vi "UTIL Temp Control.vi"(3 "Evaluate":bool, 4 "Parameters In":dbl[](array[numeric]), 5 "Class":i32) -> (1 "Parameters Out":dbl[](array[numeric]))   [LabVIEW 2010]
doc: "This VI keeps track of the number of Sleep and Wake classifications over a desired interval, and modifies the target ambient temperature based on the sleep-wake ratio. It stores 5 values in a shift register (Parameters In/Out):\n1. Error (Q - Q*)\n2. Target Temperature\n3. Sleep Count\n4. Wake Count\n5. Previous Temperature Change\n\nInputs: \n Class SGL, predicted sleep stage\n Parameters In 1-D Array of Double\n Evaluate Boolean, true at end of time period\nOutputs:\n Parameters Out 1-D Array of DBL"
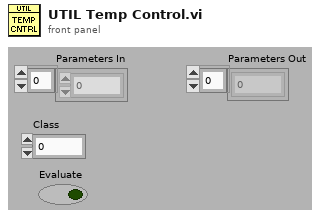
[diagram p1: front panel]
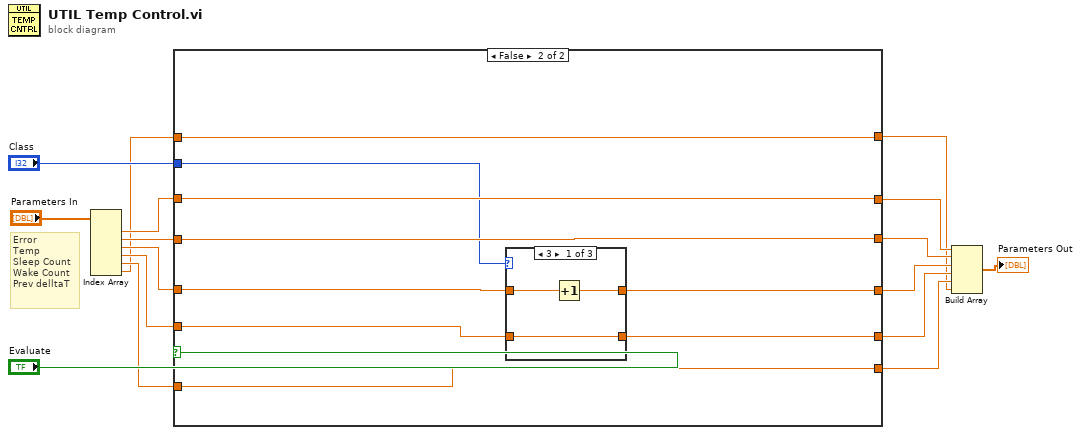
[diagram p0: block diagram]
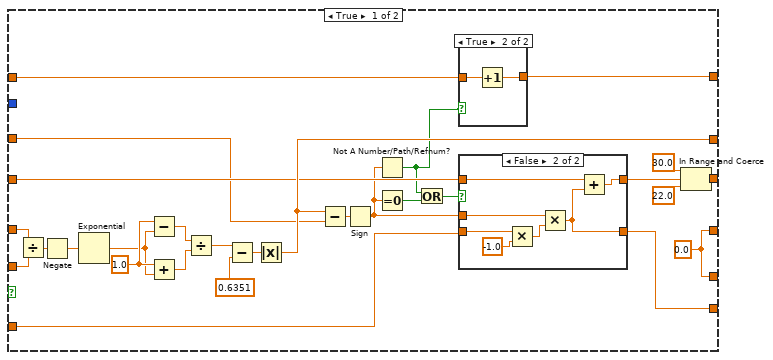
[diagram p2: hidden frame]
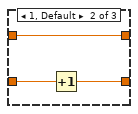
[diagram p5: hidden frame]
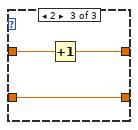
[diagram p6: hidden frame]
diagram:
  # "Error\nTemp\nSleep Count\nWake Count\nPrev delltaT"
  n1 = Index Array(array="Parameters In") -> (element #1=w8:dbl, element #2=w7:dbl, element #3=w6:dbl, element #4=w5:dbl, element #5=w3:dbl, element #6=w2:dbl)  [unwired: 6 in]
  n2 = case shown="False" "Evaluate" {
    tunnel: "Class" -> [_ w57]
    tunnel: [w44 w65] -> w12
    tunnel: w6 -> [w40 w64]
    tunnel: w5 -> [w39 w63]
    tunnel: [w44 w62] -> w11
    tunnel: w8 -> [w32 w61]
    tunnel: [w37 w61] -> w14
    tunnel: [w41 w60] -> w13
    tunnel: w7 -> [w35 w60]
    tunnel: [w36 w59] -> w4
    tunnel: w3 -> [w33 w59]
    tunnel: w2 -> [w25 w58]
    tunnel: [w24 w58] -> w1
    frame True {
      w23 = 1.0 ("x")
      w44 = 0.0
      n3 = Divide(x=w40, y=w39) -> (x/y=w22:dbl)
      n4 = Negate(x=w22) -> (-x=w21:dbl)
      n5 = Exponential(1:w21) -> (0:w20:dbl)
      n6 = Subtract(x=w23, y=w20) -> (x-y=w18:dbl)
      n7 = Add(x=w23, y=w20) -> (x+y=w17:dbl)
      n8 = Divide(x=w18, y=w17) -> (x/y=w19:dbl)
      n9 = Subtract(x=w19, y=0.6351) -> (x-y=w30:dbl)
      n10 = Absolute Value(x=w30) -> (abs(x)=w37:dbl)
      n11 = Subtract(x=w37, y=w32) -> (x-y=w38:dbl)
      n12 = Sign(1:w38) -> (0:w29:dbl)
      n13 = Not A Number/Path/Refnum?(number/path/refnum=w29) -> (NaN/Path/Refnum?=w26:bool)
      n14 = Equal To 0?(x=w29) -> (x = 0?=w28:bool)
      n15 = Or(x=w26, y=w28) -> (x .or. y?=w27:bool)
      n16 = case shown="True" w26 {
        tunnel: w25 -> [w45 w47]
        tunnel: [w45 w46] -> w24
        frame False {
        }
        frame True {
          n17 = Increment(x=w47) -> (x+1=w46:dbl)
        }
      }
      n18 = case shown="False" w27 {
        tunnel: w33 -> [w48 w51]
        tunnel: [w48 w56] -> w36
        tunnel: w35 -> [w49 w55]
        tunnel: [w49 w54] -> w34
        tunnel: w29 -> [_ w53]
        frame True {
        }
        frame False {
          n19 = Multiply(x=w51, y=-1.0) -> (x*y=w50:dbl)
          n20 = Multiply(x=w53, y=w50) -> (x*y=w56:dbl)
          n21 = Add(x=w55, y=w56) -> (x+y=w54:dbl)
        }
      }
      n22 = In Range and Coerce(upper limit=30.0 ("element"), x=w34, lower limit=22.0 ("element")) -> (coerced(x)=w41:dbl)  [unwired: 1 out]
    }
    frame False {
      n23 = case shown="3" w57 {
        tunnel: [w66 w71 w74] -> w65
        tunnel: w64 -> [w68 w71 w73]
        tunnel: w63 -> [w67 w70 w72]
        tunnel: [w67 w69 w72] -> w62
        frame 3 {
          n24 = Increment(x=w68) -> (x+1=w66:dbl)
        }
        frame 1, Default {
          n25 = Increment(x=w70) -> (x+1=w69:dbl)
        }
        frame 2 {
          n26 = Increment(x=w73) -> (x+1=w74:dbl)
        }
      }
    }
  }
  n27 = Build Array(w14, w13, w12, w11, w4, w1) -> (→"Parameters Out":dbl[])
